vi "Version_2.0_Single_Column_Code.vi"() -> ()   [LabVIEW 2020] (continued)
                            n3570 = local read "VISA Refnum in\nfor Pump"() -> (w3951:refnum<visa-resource-name>)
                            n3571 = local read "Buffer-C2 Volume \nto be Pumped"() -> (w3947:dbl)
                            n3572 = local read "Volume of Syringe"() -> (w3950:dbl)
                            n3573 = call "RPickUp(SubVI).vi"("Volume to be picked up"=w3947, "Volume of Syringe"=w3950, "Resolution of PickUP"=w3948, "PickUp Flow Rate (ul/min)"=w3949, "VISA Refnum in"=w3951) -> ()  [unwired: 6 in, 1 out]
                            n3574 = local write "SEC On"(TRUE ("SEC On")) -> ()
                          }
                          frame #22 {
                            n3575 = local read "Stopper that ends \nthe main loops"() -> (w3952:bool)
                            n3576 = local read "VISA Refnum in\nfor Pump"() -> (w3953:refnum<visa-resource-name>)
                            n3577 = case shown="True" w3952 {
                              frame False {
                              }
                              frame True {
                                n3578 = local read "VISA Refnum in\nfor Pump"() -> (w3954:refnum<visa-resource-name>)
                                n3579 = call "HardStopCurrentProcess (SubVI).vi"("VISA Refnum in"=w3954) -> ()  [unwired: 11 in]
                              }
                            }
                            n3580 = call "ProcessCompletionWaiter (SubVI).vi"("VISA Refnum in"=w3953) -> ()  [unwired: 11 in]
                          }
                          frame #23 {
                            # "Reads the initial Plunger Position for computing the volume dispensed"
                            n3581 = local read "VISA Refnum in\nfor Pump"() -> (w3956:refnum<visa-resource-name>)
                            n3582 = call "AbsolutePlungerPosition (SubVI).vi"("VISA Refnum in"=w3956) -> ("Plunger Position"=w3955:i32)  [unwired: 10 in]
                            n3583 = local write "Initial Plunger Position"(w3955) -> ()
                          }
                          frame #24 {
                            # "Switch to Port-10"
                            # "Port-10 of the pump is conncted to column-2 of chip"
                            n3584 = local read "VISA Refnum in\nfor Pump"() -> (w3958:refnum<visa-resource-name>)
                            n3585 = call "PortChanger (SubVI).vi"("Port Number"="10", "VISA Refnum in"=w3958) -> ()  [unwired: 10 in]
                          }
                          frame #25 {
                            n3586 = local read "Stopper that ends \nthe main loops"() -> (w3959:bool)
                            n3587 = local read "VISA Refnum in\nfor Pump"() -> (w3960:refnum<visa-resource-name>)
                            n3588 = case shown="True" w3959 {
                              frame False {
                              }
                              frame True {
                                n3589 = local read "VISA Refnum in\nfor Pump"() -> (w3961:refnum<visa-resource-name>)
                                n3590 = call "HardStopCurrentProcess (SubVI).vi"("VISA Refnum in"=w3961) -> ()  [unwired: 11 in]
                              }
                            }
                            n3591 = call "ProcessCompletionWaiter (SubVI).vi"("VISA Refnum in"=w3960) -> ()  [unwired: 11 in]
                          }
                          frame #26 {
                            # "Keeps the AMF valve after column-1 open and valve after column-2 closed"
                            n3592 = local read "Buffer-C2 Dispense\nFlow Rate (ul/min)"() -> (w3974:dbl)
                            n3593 = local read "Buffer-C2 Pumping\nResolution"() -> (w3973:T2)
                            n3594 = local read "VISA Refnum in\nfor Pump"() -> (w3976:refnum<visa-resource-name>)
                            n3595 = local write "Pause Data Collection"(FALSE ("Pause Data Collection")) -> ()
                            n3596 = local read "Volume of Syringe"() -> (w3975:dbl)
                            n3597 = call "GoToAbsolutePosition(SubVI).vi"("Absolute Volume Position in Syringe (in ul)"=0.0 ("Volume to be Dispensed"), "Volume of Syringe"=w3975, "Resolution of Pumping"=w3973, "Flow Rate (ul/min)"=w3974, "VISA Refnum in"=w3976) -> ()  [unwired: 6 in, 1 out]
                            n3598 = local read "VISA Refnum in\nfor Valve"() -> (w3970:refnum<visa-resource-name>)
                            n3599 = local read "External Valve \nOPEN"() -> (w3969:string)
                            n3600 = local write "Valve V1 Open"(FALSE ("Valve V1 Open")) -> ()
                            n3601 = local write "Valve V2 Open"(TRUE ("Valve V2 Open")) -> ()
                            n3602 = local write "Valve V3 Open"(TRUE ("Valve V3 Open")) -> ()
                            n3603 = local write "Valve V4 Open"(FALSE ("Valve V4 Open")) -> ()
                            n3604 = call "PortChanger_Valve (SubVI).vi"("Port Number"=w3969, "VISA Refnum in"=w3970) -> ()  [unwired: 10 in]
                            n3605 = local write "Valve V5 Open"(FALSE ("Valve V5 Open")) -> ()
                            n3606 = local write "Valve V6 Open"(FALSE ("Valve V6 Open")) -> ()
                            n3607 = local write "Valve V7 Open"(FALSE ("Valve V7 Open")) -> ()
                          }
                          frame #27 {
                            n3608 = local read "Initial Plunger Position"() -> (w3980:dbl)
                            n3609 = local read "Buffer-C2 Pumping\nResolution"() -> (w3979:T2)
                            n3610 = local read "VISA Refnum in\nfor Pump"() -> (w3981:refnum<visa-resource-name>)
                            n3611 = local read "Volume of Syringe"() -> (w3978:dbl)
                            n3612 = while {
                              tunnel: w3980 -> [w3987]
                              tunnel: w3981 -> [w3986]
                              tunnel: w3979 -> [w3985]
                              tunnel: w3978 -> [w3984]
                              stop <- w3982 stop-if-true
                              n3613 = Wait (ms)(milliseconds to wait=u32 100) -> ()  [unwired: 1 out]
                              n3614 = stacked-sequence {
                                tunnel: w3987 -> [w3993 _]
                                tunnel: w3986 -> [w3992 w4019]
                                tunnel: w3985 -> [w3991 _]
                                tunnel: w3984 -> [w3990 _]
                                tunnel: [_ w4015] -> w3982
                                frame #0 {
                                n3615 = call "AbsolutePlungerPosition (SubVI).vi"("VISA Refnum in"=w3992) -> ("Plunger Position"=w3989:i32)  [unwired: 10 in]
                                n3616 = case shown="\"Standard Pumping\", Default" w3991 {
                                tunnel: w3993 -> [w3998 w4007]
                                tunnel: w3989 -> [w3999 w4006]
                                tunnel: [w3997 w4004] -> w3988
                                tunnel: w3990 -> [w3996 w4005]
                                frame "Standard Pumping", Default {
                                n3617 = Subtract(x=w3998, y=w3999) -> (x-y=w3995:dbl)
                                n3618 = Absolute Value(x=w3995) -> (abs(x)=w3994:dbl)
                                n3619 = Multiply(x=w3994, y=w3996) -> (x*y=w4001:dbl)
                                n3620 = Divide(x=w4001, y=3000.0) -> (x/y=w3997:dbl)
                                }
                                frame "High Resolution Pumping" {
                                n3621 = Subtract(x=w4007, y=w4006) -> (x-y=w4003:dbl)
                                n3622 = Absolute Value(x=w4003) -> (abs(x)=w4002:dbl)
                                n3623 = Multiply(x=w4002, y=w4005) -> (x*y=w4009:dbl)
                                n3624 = Divide(x=w4009, y=24000.0) -> (x/y=w4004:dbl)
                                }
                                }
                                n3625 = local write "Volume being Injected \nin this process"(w3988) -> ()
                                }
                                frame #1 {
                                n3626 = local read "Stopper that ends \nthe main loops"() -> (w4016:bool)
                                n3627 = local read "Divert Buffer-C \ninto Column-2"() -> (w4017:bool)
                                n3628 = local read "Volume being Injected \nin this process"() -> (w4014:dbl)
                                n3629 = call "LSPOneStatus (SubVI).vi"("VISA Refnum in"=w4019) -> ("read buffer"=w4021:string)  [unwired: 10 in]
                                n3630 = call <vilib>:"Trim Whitespace.vi"("string"=w4021) -> ("trimmed string"=w4020:string)  [unwired: 1 in]
                                n3631 = Equal?(x=w4020, y="/0`\u0003") -> (x = y?=w4018:bool)
                                n3632 = Or(x=w4017, y=w4016) -> (x .or. y?=w4012:bool)
                                n3633 = Greater Or Equal?(x=w4014, y=2.0) -> (x >= y?=w4011:bool)
                                n3634 = Or(x=w4012, y=w4011) -> (x .or. y?=w4010:bool)
                                n3635 = Or(x=w4018, y=w4010) -> (x .or. y?=w4015:bool)
                                }
                              }
                            }
                            n3636 = local read "Stopper that ends \nthe main loops"() -> (w3977:bool)
                            n3637 = case shown="True" w3977 {
                              frame False {
                              }
                              frame True {
                                n3638 = local read "VISA Refnum in\nfor Pump"() -> (w4023:refnum<visa-resource-name>)
                                n3639 = call "HardStopCurrentProcess (SubVI).vi"("VISA Refnum in"=w4023) -> ()  [unwired: 11 in]
                              }
                            }
                          }
                          frame #28 {
                            # "Keeps the on-chip valves V4, V5 and V7 open"
                            # "Keeps the AMF valve after column-1 closed and valve after column-2 open"
                            n3640 = local write "Divert Buffer-C \ninto Column-2"(FALSE ("Divert Buffer-C \ninto Column-2")) -> ()
                            n3641 = local read "VISA Refnum in\nfor Pump"() -> (w4028:refnum<visa-resource-name>)
                            n3642 = local read "External Valve \nCLOSED"() -> (w4027:string)
                            n3643 = local write "Valve V3 Open"(FALSE ("Valve V3 Open")) -> ()
                            n3644 = local write "Valve V2 Open"(FALSE ("Valve V2 Open")) -> ()
                            n3645 = local write "Valve V1 Open"(FALSE ("Valve V1 Open")) -> ()
                            n3646 = local write "Valve V4 Open"(TRUE ("Valve V4 Open")) -> ()
                            n3647 = call "PortChanger_Valve (SubVI).vi"("Port Number"=w4027, "VISA Refnum in"=w4028) -> ()  [unwired: 10 in]
                            n3648 = local write "Valve V5 Open"(TRUE ("Valve V5 Open")) -> ()
                            n3649 = local write "Valve V6 Open"(FALSE ("Valve V6 Open")) -> ()
                            n3650 = local write "Valve V7 Open"(TRUE ("Valve V7 Open")) -> ()
                          }
                          frame #29 {
                            n3651 = local read "Initial Plunger Position"() -> (w4037:dbl)
                            n3652 = local read "Buffer-C2 Pumping\nResolution"() -> (w4036:T2)
                            n3653 = local read "VISA Refnum in\nfor Pump"() -> (w4038:refnum<visa-resource-name>)
                            n3654 = local read "Volume of Syringe"() -> (w4035:dbl)
                            n3655 = while {
                              tunnel: w4037 -> [w4044]
                              tunnel: w4038 -> [w4043]
                              tunnel: w4036 -> [w4042]
                              tunnel: w4035 -> [w4041]
                              stop <- w4039 stop-if-true
                              n3656 = Wait (ms)(milliseconds to wait=u32 100) -> ()  [unwired: 1 out]
                              n3657 = stacked-sequence {
                                tunnel: w4044 -> [w4050 _]
                                tunnel: w4043 -> [w4049 w4072]
                                tunnel: w4042 -> [w4048 _]
                                tunnel: w4041 -> [w4047 _]
                                tunnel: [_ w4070] -> w4039
                                frame #0 {
                                n3658 = call "AbsolutePlungerPosition (SubVI).vi"("VISA Refnum in"=w4049) -> ("Plunger Position"=w4046:i32)  [unwired: 10 in]
                                n3659 = case shown="\"Standard Pumping\", Default" w4048 {
                                tunnel: w4050 -> [w4055 w4064]
                                tunnel: w4046 -> [w4056 w4063]
                                tunnel: [w4054 w4061] -> w4045
                                tunnel: w4047 -> [w4053 w4062]
                                frame "Standard Pumping", Default {
                                n3660 = Subtract(x=w4055, y=w4056) -> (x-y=w4052:dbl)
                                n3661 = Absolute Value(x=w4052) -> (abs(x)=w4051:dbl)
                                n3662 = Multiply(x=w4051, y=w4053) -> (x*y=w4058:dbl)
                                n3663 = Divide(x=w4058, y=3000.0) -> (x/y=w4054:dbl)
                                }
                                frame "High Resolution Pumping" {
                                n3664 = Subtract(x=w4064, y=w4063) -> (x-y=w4060:dbl)
                                n3665 = Absolute Value(x=w4060) -> (abs(x)=w4059:dbl)
                                n3666 = Multiply(x=w4059, y=w4062) -> (x*y=w4066:dbl)
                                n3667 = Divide(x=w4066, y=24000.0) -> (x/y=w4061:dbl)
                                }
                                }
                                n3668 = local write "Volume being Injected \nin this process"(w4045) -> ()
                                }
                                frame #1 {
                                n3669 = call "LSPOneStatus (SubVI).vi"("VISA Refnum in"=w4072) -> ("read buffer"=w4074:string)  [unwired: 10 in]
                                n3670 = call <vilib>:"Trim Whitespace.vi"("string"=w4074) -> ("trimmed string"=w4073:string)  [unwired: 1 in]
                                n3671 = Equal?(x=w4073, y="/0`\u0003") -> (x = y?=w4071:bool)
                                n3672 = local read "Stopper that ends \nthe main loops"() -> (w4068:bool)
                                n3673 = local read "Divert Sample \nonto Grid"() -> (w4069:bool)
                                n3674 = Or(x=w4069, y=w4068) -> (x .or. y?=w4067:bool)
                                n3675 = Or(x=w4071, y=w4067) -> (x .or. y?=w4070:bool)
                                }
                              }
                            }
                            n3676 = local read "Stopper that ends \nthe main loops"() -> (w4034:bool)
                            n3677 = case shown="True" w4034 {
                              frame False {
                              }
                              frame True {
                                n3678 = local read "VISA Refnum in\nfor Pump"() -> (w4076:refnum<visa-resource-name>)
                                n3679 = call "HardStopCurrentProcess (SubVI).vi"("VISA Refnum in"=w4076) -> ()  [unwired: 11 in]
                              }
                            }
                          }
                          frame #30 {
                            n3680 = local read "Volume being Injected \nin this process"() -> (w4079:dbl)
                            n3681 = local read "VISA Refnum in\nfor Pump"() -> (w4081:refnum<visa-resource-name>)
                            n3682 = call "AbsolutePlungerPosition (SubVI).vi"("VISA Refnum in"=w4081) -> ("Plunger Position"=w4080:i32)  [unwired: 10 in]
                            n3683 = local write "Pause Data Collection"(TRUE) -> ()
                            n3684 = local write "True Volume being \ninjected in this\nprocess"(w4079) -> ()
                            n3685 = local write "Position\nNow"(w4080) -> ()
                            n3686 = Wait (ms)(milliseconds to wait=u32 500) -> ()  [unwired: 1 out]
                          }
                          frame #31 {
                            # "Sample Deposition onto EM-Grid"
                            n3687 = local read "Divert Sample \nonto Grid"() -> (w4082:bool)
                            n3688 = case shown="True" w4082 {
                              frame False {
                              }
                              frame True {
                                n3689 = stacked-sequence {
                                frame #0 {
                                # "Discard the initial volume of fluid that is present in the channel prior to detection"
                                n3690 = local read "Buffer-C2 Pumping\nResolution"() -> (w4093:T2)
                                n3691 = local read "Initial Plunger Position"() -> (w4092:dbl)
                                n3692 = local read "VISA Refnum in\nfor Pump"() -> (w4094:refnum<visa-resource-name>)
                                n3693 = local read "Position\nNow"() -> (w4090:dbl)
                                n3694 = local read "Volume of Syringe"() -> (w4091:dbl)
                                n3695 = local write "Pause Data Collection"(FALSE) -> ()
                                n3696 = while {
                                tunnel: w4094 -> [w4104]
                                tunnel: w4093 -> [w4103]
                                tunnel: w4092 -> [w4099]
                                tunnel: w4091 -> [w4102]
                                tunnel: w4090 -> [w4098]
                                stop <- w4100 stop-if-true
                                n3697 = stacked-sequence {
                                tunnel: w4104 -> [w4110 w4132 w4162]
                                tunnel: w4103 -> [w4109 w4131 _]
                                tunnel: w4099 -> [w4107 _ _]
                                tunnel: w4102 -> [w4106 w4129 _]
                                tunnel: [_ _ w4155] -> w4100
                                tunnel: w4098 -> [_ w4127 _]
                                frame #0 {
                                # "From here on 'True Volume being injected \nin this process' represents the true total \nvolume in this process"
                                n3698 = call "AbsolutePlungerPosition (SubVI).vi"("VISA Refnum in"=w4110) -> ("Plunger Position"=w4108:i32)  [unwired: 10 in]
                                n3699 = case shown="..\"Standard Pumping\"" w4109 {
                                tunnel: w4108 -> [w4118 w4126]
                                tunnel: w4107 -> [w4117 w4125]
                                tunnel: w4106 -> [w4114 w4122]
                                tunnel: [w4111 w4119] -> w4105
                                frame .."Standard Pumping" {
                                n3700 = Subtract(x=w4118, y=w4117) -> (x-y=w4116:dbl)
                                n3701 = Absolute Value(x=w4116) -> (abs(x)=w4115:dbl)
                                n3702 = Multiply(x=w4115, y=w4114) -> (x*y=w4113:dbl)
                                n3703 = Divide(x=w4113, y=3000.0) -> (x/y=w4111:dbl)
                                }
                                frame "High Resolution Pumping".. {
                                n3704 = Subtract(x=w4126, y=w4125) -> (x-y=w4124:dbl)
                                n3705 = Absolute Value(x=w4124) -> (abs(x)=w4123:dbl)
                                n3706 = Multiply(x=w4123, y=w4122) -> (x*y=w4121:dbl)
                                n3707 = Divide(x=w4121, y=24000.0) -> (x/y=w4119:dbl)
                                }
                                }
                                n3708 = local write "True Volume being \ninjected in this\nprocess"(w4105) -> ()
                                }
                                frame #1 {
                                # "From here on 'Volume being injected \nin this process' represents the volume \nin this sub process"
                                n3709 = call "AbsolutePlungerPosition (SubVI).vi"("VISA Refnum in"=w4132) -> ("Plunger Position"=w4130:i32)  [unwired: 10 in]
                                n3710 = case shown="..\"Standard Pumping\"" w4131 {
                                tunnel: w4130 -> [w4140 w4148]
                                tunnel: w4127 -> [w4139 w4147]
                                tunnel: w4129 -> [w4136 w4144]
                                tunnel: [w4133 w4141] -> w4128
                                frame .."Standard Pumping" {
                                n3711 = Subtract(x=w4140, y=w4139) -> (x-y=w4138:dbl)
                                n3712 = Absolute Value(x=w4138) -> (abs(x)=w4137:dbl)
                                n3713 = Multiply(x=w4137, y=w4136) -> (x*y=w4135:dbl)
                                n3714 = Divide(x=w4135, y=3000.0) -> (x/y=w4133:dbl)
                                }
                                frame "High Resolution Pumping".. {
                                n3715 = Subtract(x=w4148, y=w4147) -> (x-y=w4146:dbl)
                                n3716 = Absolute Value(x=w4146) -> (abs(x)=w4145:dbl)
                                n3717 = Multiply(x=w4145, y=w4144) -> (x*y=w4143:dbl)
                                n3718 = Divide(x=w4143, y=24000.0) -> (x/y=w4141:dbl)
                                }
                                }
                                n3719 = local write "Volume being Injected \nin this process"(w4128) -> ()
                                }
                                frame #2 {
                                n3720 = local read "Discard Volume"() -> (w4149:dbl)
                                n3721 = local read "Discard fluid \nprior to 1st \ndeposition"() -> (w4154:bool)
                                n3722 = local read "Volume being Injected \nin this process"() -> (w4153:dbl)
                                n3723 = Greater Or Equal?(x=w4153, y=w4149) -> (x >= y?=w4151:bool)
                                n3724 = call "AbsolutePlungerPositionStatus (SubVI).vi"("VISA Refnum in"=w4162) -> ("read buffer"=w4161:string)  [unwired: 10 in]
                                n3725 = local read "Stop for End of \nExperiment \nand Data Writing"() -> (w4158:bool)
                                n3726 = call <vilib>:"Trim Whitespace.vi"("string"=w4161) -> ("trimmed string"=w4160:string)  [unwired: 1 in]
                                n3727 = Not(x=w4154) -> (.not. x?=w4152:bool)
                                n3728 = Equal?(x=w4160, y="/0`\u0003") -> (x = y?=w4157:bool)
                                n3729 = Or(x=w4152, y=w4151) -> (x .or. y?=w4150:bool)
                                n3730 = Or(x=w4150, y=w4158) -> (x .or. y?=w4156:bool)
                                n3731 = Or(x=w4157, y=w4156) -> (x .or. y?=w4155:bool)
                                }
                                }
                                n3732 = Wait (ms)(milliseconds to wait=u32 100) -> ()  [unwired: 1 out]
                                }
                                n3733 = local write "Valve V4 Open"(TRUE ("Valve V4 Open")) -> ()
                                n3734 = local write "Valve V3 Open"(FALSE ("Valve V3 Open")) -> ()
                                n3735 = local write "Valve V2 Open"(FALSE ("Valve V2 Open")) -> ()
                                n3736 = local write "Valve V1 Open"(FALSE ("Valve V1 Open")) -> ()
                                n3737 = local write "Valve V5 Open"(TRUE ("Valve V5 Open")) -> ()
                                n3738 = local write "Valve V6 Open"(TRUE ("Valve V6 Open")) -> ()
                                n3739 = local write "Valve V7 Open"(FALSE ("Valve V7 Open")) -> ()
                                n3740 = local write "Volume being Injected \nin this process"(0.0) -> ()
                                }
                                frame #1 {
                                # "Keeps the on-chip valve V1, V2 and V3 closed,\nHalts also deposition onto the grid\nand waits for the 1st redeposit command. Once the command is issued\nit starts pumpoing and moves onto the next frame"
                                n3741 = stacked-sequence {
                                frame #0 {
                                n3742 = local write "Valve V5 Open"(FALSE ("Valve V5 Open")) -> ()
                                n3743 = local write "Valve V1 Open"(FALSE ("Valve V1 Open")) -> ()
                                n3744 = local read "VISA Refnum in\nfor Pump"() -> (w4172:refnum<visa-resource-name>)
                                n3745 = local write "Valve V2 Open"(FALSE ("Valve V2 Open")) -> ()
                                n3746 = local write "Valve V6 Open"(FALSE ("Valve V6 Open")) -> ()
                                n3747 = local write "Re-deposit Sample\nonto Grid"(FALSE ("Redeposit Sample\nonto Grid")) -> ()
                                n3748 = local write "Pause Data Collection"(TRUE ("Pause Data Collection")) -> ()
                                n3749 = call "HardStopCurrentProcess (SubVI).vi"("VISA Refnum in"=w4172) -> ()  [unwired: 11 in]
                                n3750 = local write "Valve V7 Open"(FALSE ("Valve V7 Open")) -> ()
                                n3751 = local write "Valve V3 Open"(FALSE ("Valve V3 Open")) -> ()
                                n3752 = local write "Valve V4 Open"(FALSE ("Valve V4 Open")) -> ()
                                }
                                frame #1 {
                                n3753 = while {
                                stop <- w4175 stop-if-true
                                n3754 = local read "Stop for End of \nExperiment \nand Data Writing"() -> (w4176:bool)
                                n3755 = local read "Re-deposit Sample\nonto Grid"() -> (w4177:bool)
                                n3756 = Or(x=w4177, y=w4176) -> (x .or. y?=w4175:bool)
                                }
                                n3757 = local write "Discard fluid \nprior to 1st \ndeposition"(FALSE ("Discard fluid \nprior to 1st \ndeposition")) -> ()
                                n3758 = One Button Dialog(message="Do you want to deposit sample on another grid? If yes, turn on 'Re-deposit Sample onto Grid'. Else turn on STOP ") -> ()  [unwired: 1 in, 1 out]
                                }
                                frame #2 {
                                n3759 = local write "Valve V6 Open"(TRUE ("Valve V3 Open")) -> ()
                                n3760 = local write "Valve V4 Open"(TRUE ("Valve V1 Open")) -> ()
                                n3761 = local write "Valve V5 Open"(TRUE ("Valve V2 Open")) -> ()
                                n3762 = local write "Valve V7 Open"(FALSE ("Valve V7 Open")) -> ()
                                }
                                frame #3 {
                                n3763 = local read "Re-deposit Sample\nonto Grid"() -> (w4182:bool)
                                n3764 = case shown="True" w4182 {
                                frame False {
                                n3765 = local write "Suction On/Off"(FALSE ("Suction On/Off")) -> ()
                                }
                                frame True {
                                n3766 = stacked-sequence {
                                frame #0 {
                                n3767 = local read "VISA Refnum in\nfor Pump"() -> (w4185:refnum<visa-resource-name>)
                                n3768 = call "AbsolutePlungerPosition (SubVI).vi"("VISA Refnum in"=w4185) -> ("Plunger Position"=w4184:i32)  [unwired: 10 in]
                                n3769 = local write "Position\nNow"(w4184) -> ()
                                }
                                frame #1 {
                                n3770 = local read "Buffer-C2 Pumping\nResolution"() -> (w4187:T2)
                                n3771 = case shown="\"Standard Pumping\", Default" w4187 {
                                tunnel: [w4188 w4199] -> w4186
                                frame "Standard Pumping", Default {
                                n3772 = local read "Buffer-C2 Volume \nto be Pumped"() -> (w4191:dbl)
                                n3773 = local read "Volume of Syringe"() -> (w4194:dbl)
                                n3774 = local read "Initial Plunger Position"() -> (w4198:dbl)
                                n3775 = local read "Position\nNow"() -> (w4197:dbl)
                                n3776 = Subtract(x=w4198, y=w4197) -> (x-y=w4196:dbl)
                                n3777 = Absolute Value(x=w4196) -> (abs(x)=w4195:dbl)
                                n3778 = Multiply(x=w4195, y=w4194) -> (x*y=w4193:dbl)
                                n3779 = Divide(x=w4193, y=3000.0) -> (x/y=w4190:dbl)
                                n3780 = Subtract(x=w4190, y=w4191) -> (x-y=w4189:dbl)
                                n3781 = Absolute Value(x=w4189) -> (abs(x)=w4188:dbl)
                                }
                                frame "High Resolution Pumping" {
                                n3782 = local read "Buffer-C2 Volume \nto be Pumped"() -> (w4202:dbl)
                                n3783 = local read "Volume of Syringe"() -> (w4205:dbl)
                                n3784 = local read "Initial Plunger Position"() -> (w4209:dbl)
                                n3785 = local read "Position\nNow"() -> (w4208:dbl)
                                n3786 = Subtract(x=w4209, y=w4208) -> (x-y=w4207:dbl)
                                n3787 = Absolute Value(x=w4207) -> (abs(x)=w4206:dbl)
                                n3788 = Multiply(x=w4206, y=w4205) -> (x*y=w4204:dbl)
                                n3789 = Divide(x=w4204, y=24000.0) -> (x/y=w4201:dbl)
                                n3790 = Subtract(x=w4201, y=w4202) -> (x-y=w4200:dbl)
                                n3791 = Absolute Value(x=w4200) -> (abs(x)=w4199:dbl)
                                }
                                }
                                n3792 = local write "Buffer-C Volume\nleft to be Pumped"(w4186) -> ()
                                }
                                frame #2 {
                                n3793 = local read "Buffer-C2 Dispense\nFlow Rate (ul/min)"() -> (w4213:dbl)
                                n3794 = local read "Buffer-C2 Pumping\nResolution"() -> (w4212:T2)
                                n3795 = local read "VISA Refnum in\nfor Pump"() -> (w4215:refnum<visa-resource-name>)
                                n3796 = local read "Volume of Syringe"() -> (w4214:dbl)
                                n3797 = call "GoToAbsolutePosition(SubVI).vi"("Absolute Volume Position in Syringe (in ul)"=0.0, "Volume of Syringe"=w4214, "Resolution of Pumping"=w4212, "Flow Rate (ul/min)"=w4213, "VISA Refnum in"=w4215) -> ()  [unwired: 6 in, 1 out]
                                n3798 = local write "Suction On/Off"(FALSE ("Suction On/Off")) -> ()
                                }
                                }
                                }
                                }
                                }
                                frame #4 {
                                n3799 = local read "Stop for End of \nExperiment \nand Data Writing"() -> (w4216:bool)
                                n3800 = case shown="True" w4216 {
                                frame False {
                                }
                                frame True {
                                n3801 = local read "VISA Refnum in\nfor Pump"() -> (w4217:refnum<visa-resource-name>)
                                n3802 = call "HardStopCurrentProcess (SubVI).vi"("VISA Refnum in"=w4217) -> ()  [unwired: 11 in]
                                }
                                }
                                }
                                }
                                }
                                frame #2 {
                                # "Keeps the on-chip valve V1, V2 Open and V3 closed"
                                n3803 = while {
                                stop <- w4221 stop-if-true
                                n3804 = local read "Suction On/Off"() -> (w4222:bool)
                                n3805 = case shown="True" w4222 {
                                frame False {
                                n3806 = local read "Buffer-C2 Pumping\nResolution"() -> (w4228:T2)
                                n3807 = local read "Initial Plunger Position"() -> (w4227:dbl)
                                n3808 = local read "VISA Refnum in\nfor Pump"() -> (w4229:refnum<visa-resource-name>)
                                n3809 = local read "Position\nNow"() -> (w4225:dbl)
                                n3810 = local read "Volume of Syringe"() -> (w4226:dbl)
                                n3811 = local write "Volume being Injected \nin this process"(0.0) -> ()
                                n3812 = local write "Pause Data Collection"(FALSE) -> ()
                                n3813 = while {
                                tunnel: w4229 -> [w4236]
                                tunnel: w4228 -> [w4235]
                                tunnel: w4227 -> [w4231]
                                tunnel: w4226 -> [w4234]
                                tunnel: w4225 -> [w4230]
                                stop <- w4232 stop-if-true
                                n3814 = stacked-sequence {
                                tunnel: w4236 -> [w4242 w4264 w4289]
                                tunnel: w4235 -> [w4241 w4263 _]
                                tunnel: w4231 -> [w4239 _ _]
                                tunnel: w4234 -> [w4238 w4261 _]
                                tunnel: [_ _ w4281] -> w4232
                                tunnel: w4230 -> [_ w4259 _]
                                frame #0 {
                                # "From here on 'True Volume being injected \nin this process' represents the true total \nvolume in this process"
                                n3815 = call "AbsolutePlungerPosition (SubVI).vi"("VISA Refnum in"=w4242) -> ("Plunger Position"=w4240:i32)  [unwired: 10 in]
                                n3816 = case shown="..\"Standard Pumping\"" w4241 {
                                tunnel: w4240 -> [w4250 w4258]
                                tunnel: w4239 -> [w4249 w4257]
                                tunnel: w4238 -> [w4246 w4254]
                                tunnel: [w4243 w4251] -> w4237
                                frame .."Standard Pumping" {
                                n3817 = Subtract(x=w4250, y=w4249) -> (x-y=w4248:dbl)
                                n3818 = Absolute Value(x=w4248) -> (abs(x)=w4247:dbl)
                                n3819 = Multiply(x=w4247, y=w4246) -> (x*y=w4245:dbl)
                                n3820 = Divide(x=w4245, y=3000.0) -> (x/y=w4243:dbl)
                                }
                                frame "High Resolution Pumping".. {
                                n3821 = Subtract(x=w4258, y=w4257) -> (x-y=w4256:dbl)
                                n3822 = Absolute Value(x=w4256) -> (abs(x)=w4255:dbl)
                                n3823 = Multiply(x=w4255, y=w4254) -> (x*y=w4253:dbl)
                                n3824 = Divide(x=w4253, y=24000.0) -> (x/y=w4251:dbl)
                                }
                                }
                                n3825 = local write "True Volume being \ninjected in this\nprocess"(w4237) -> ()
                                }
                                frame #1 {
                                # "From here on 'Volume being injected \nin this process' represents the volume \nin this sub process"
                                n3826 = call "AbsolutePlungerPosition (SubVI).vi"("VISA Refnum in"=w4264) -> ("Plunger Position"=w4262:i32)  [unwired: 10 in]
                                n3827 = case shown="..\"Standard Pumping\"" w4263 {
                                tunnel: w4262 -> [w4272 w4280]
                                tunnel: w4259 -> [w4271 w4279]
                                tunnel: w4261 -> [w4268 w4276]
                                tunnel: [w4265 w4273] -> w4260
                                frame .."Standard Pumping" {
                                n3828 = Subtract(x=w4272, y=w4271) -> (x-y=w4270:dbl)
                                n3829 = Absolute Value(x=w4270) -> (abs(x)=w4269:dbl)
                                n3830 = Multiply(x=w4269, y=w4268) -> (x*y=w4267:dbl)
                                n3831 = Divide(x=w4267, y=3000.0) -> (x/y=w4265:dbl)
                                }
                                frame "High Resolution Pumping".. {
                                n3832 = Subtract(x=w4280, y=w4279) -> (x-y=w4278:dbl)
                                n3833 = Absolute Value(x=w4278) -> (abs(x)=w4277:dbl)
                                n3834 = Multiply(x=w4277, y=w4276) -> (x*y=w4275:dbl)
                                n3835 = Divide(x=w4275, y=24000.0) -> (x/y=w4273:dbl)
                                }
                                }
                                n3836 = local write "Volume being Injected \nin this process"(w4260) -> ()
                                }
                                frame #2 {
                                n3837 = local read "Stop for End of \nExperiment \nand Data Writing"() -> (w4284:bool)
                                n3838 = local read "Suction On/Off"() -> (w4285:bool)
                                n3839 = call "AbsolutePlungerPositionStatus (SubVI).vi"("VISA Refnum in"=w4289) -> ("read buffer"=w4288:string)  [unwired: 10 in]
                                n3840 = call <vilib>:"Trim Whitespace.vi"("string"=w4288) -> ("trimmed string"=w4287:string)  [unwired: 1 in]
                                n3841 = Equal?(x=w4287, y="/0`\u0003") -> (x = y?=w4283:bool)
                                n3842 = Or(x=w4285, y=w4284) -> (x .or. y?=w4282:bool)
                                n3843 = Or(x=w4283, y=w4282) -> (x .or. y?=w4281:bool)
                                }
                                }
                                n3844 = Wait (ms)(milliseconds to wait=u32 100) -> ()  [unwired: 1 out]
                                }
                                }
                                frame True {
                                n3845 = stacked-sequence {
                                frame #0 {
                                n3846 = local read "Suction Pressure\nfor EM-grid \nDeposition (mbar)"() -> (w4294:sgl)
                                n3847 = local write "Valve V4 Open"(FALSE ("Valve V4 Open")) -> ()
                                n3848 = local read "VISA Refnum in\nfor Pump"() -> (w4297:refnum<visa-resource-name>)
                                n3849 = local write "Valve V5 Open"(FALSE ("Valve V1 Open")) -> ()
                                n3850 = local write "Suction pressure \nfor grid deposition"(w4294) -> ()
                                n3851 = local write "Re-deposit Sample\nonto Grid"(FALSE ("Redeposit Sample\nonto Grid")) -> ()
                                n3852 = local write "Pause Data Collection"(TRUE ("Pause Data Collection")) -> ()
                                n3853 = call "HardStopCurrentProcess (SubVI).vi"("VISA Refnum in"=w4297) -> ()  [unwired: 11 in]
                                n3854 = local write "Valve V6 Open"(TRUE ("Valve V2 Open")) -> ()
                                n3855 = local write "Valve V7 Open"(TRUE ("Valve V3 Open")) -> ()
                                }
                                frame #1 {
                                n3856 = call <vilib>:"fgt init.vi"() -> ("error out"=w4298:errorcluster)  [unwired: 11 in]
                                n3857 = while {
                                tunnel: [w4302] -> w4299
                                tunnel: w4298 -> [w4301]
                                stop <- w4305 stop-if-true
                                # "'5' corresponds to 2nd positin in the line-up series"
                                n3858 = local read "Suction On/Off"() -> (w4300:bool)
                                n3859 = local read "Stop for End of \nExperiment \nand Data Writing"() -> (w4306:bool)
                                n3860 = case shown="True" w4300 {
                                tunnel: [0 w4311] -> w4303
                                frame False {
                                }
                                frame True {
                                n3861 = local read "Suction Pressure\nfor EM-grid \nDeposition (mbar)"() -> (w4311:sgl)
                                }
                                }
                                n3862 = call <vilib>:"fgt set pressure.vi"("error in (no error)"=w4301, "pressure"=w4303, "pressureIndex"=u32 1) -> ("error out"=w4302:errorcluster)  [unwired: 8 in]
                                n3863 = local read "Suction On/Off"() -> (w4308:bool)
                                n3864 = Not(x=w4308) -> (.not. x?=w4307:bool)
                                n3865 = Wait (ms)(milliseconds to wait=u32 100) -> ()  [unwired: 1 out]
                                n3866 = Or(x=w4307, y=w4306) -> (x .or. y?=w4305:bool)
                                }
                                n3867 = call <vilib>:"fgt close.vi"("error in (no error)"=w4299) -> ()  [unwired: 10 in, 1 out]
                                }
                                frame #2 {
                                n3868 = local write "Valve V7 Open"(FALSE ("Valve V3 Open")) -> ()
                                n3869 = local write "Valve V5 Open"(FALSE ("Valve V1 Open")) -> ()
                                n3870 = local write "Valve V6 Open"(FALSE ("Valve V2 Open")) -> ()
                                n3871 = local write "Valve V4 Open"(FALSE ("Valve V4 Open")) -> ()
                                }
                                frame #3 {
                                n3872 = while {
                                stop <- w4317 stop-if-true
                                n3873 = local read "Stop for End of \nExperiment \nand Data Writing"() -> (w4318:bool)
                                n3874 = local read "Re-deposit Sample\nonto Grid"() -> (w4319:bool)
                                n3875 = Or(x=w4319, y=w4318) -> (x .or. y?=w4317:bool)
                                }
                                n3876 = One Button Dialog(message="Do you want to deposit sample on another grid? If yes, turn on 'Re-deposit Sample onto Grid'. Else turn on STOP ") -> ()  [unwired: 1 in, 1 out]
                                }
                                frame #4 {
                                n3877 = local write "Valve V4 Open"(TRUE ("Valve V4 Open")) -> ()
                                n3878 = local write "Valve V7 Open"(FALSE ("Valve V3 Open")) -> ()
                                n3879 = local write "Valve V5 Open"(TRUE ("Valve V1 Open")) -> ()
                                n3880 = local write "Valve V6 Open"(TRUE ("Valve V2 Open")) -> ()
                                }
                                frame #5 {
                                n3881 = local read "Re-deposit Sample\nonto Grid"() -> (w4324:bool)
                                n3882 = case shown="False" w4324 {
                                frame False {
                                n3883 = local write "Suction On/Off"(FALSE ("Suction On/Off")) -> ()
                                }
                                frame True {
                                n3884 = stacked-sequence {
                                frame #0 {
                                n3885 = local read "VISA Refnum in\nfor Pump"() -> (w4327:refnum<visa-resource-name>)
                                n3886 = call "AbsolutePlungerPosition (SubVI).vi"("VISA Refnum in"=w4327) -> ("Plunger Position"=w4326:i32)  [unwired: 10 in]
                                n3887 = local write "Position\nNow"(w4326) -> ()
                                }
                                frame #1 {
                                n3888 = local read "Buffer-C2 Pumping\nResolution"() -> (w4329:T2)
                                n3889 = case shown="\"Standard Pumping\", Default" w4329 {
                                tunnel: [w4330 w4341] -> w4328
                                frame "Standard Pumping", Default {
                                n3890 = local read "Buffer-C2 Volume \nto be Pumped"() -> (w4333:dbl)
                                n3891 = local read "Volume of Syringe"() -> (w4336:dbl)
                                n3892 = local read "Initial Plunger Position"() -> (w4340:dbl)
                                n3893 = local read "Position\nNow"() -> (w4339:dbl)
                                n3894 = Subtract(x=w4340, y=w4339) -> (x-y=w4338:dbl)
                                n3895 = Absolute Value(x=w4338) -> (abs(x)=w4337:dbl)
                                n3896 = Multiply(x=w4337, y=w4336) -> (x*y=w4335:dbl)
                                n3897 = Divide(x=w4335, y=3000.0) -> (x/y=w4332:dbl)
                                n3898 = Subtract(x=w4332, y=w4333) -> (x-y=w4331:dbl)
                                n3899 = Absolute Value(x=w4331) -> (abs(x)=w4330:dbl)
                                }
                                frame "High Resolution Pumping" {
                                n3900 = local read "Buffer-C2 Volume \nto be Pumped"() -> (w4344:dbl)
                                n3901 = local read "Volume of Syringe"() -> (w4347:dbl)
                                n3902 = local read "Initial Plunger Position"() -> (w4351:dbl)
                                n3903 = local read "Position\nNow"() -> (w4350:dbl)
                                n3904 = Subtract(x=w4351, y=w4350) -> (x-y=w4349:dbl)
                                n3905 = Absolute Value(x=w4349) -> (abs(x)=w4348:dbl)
                                n3906 = Multiply(x=w4348, y=w4347) -> (x*y=w4346:dbl)
                                n3907 = Divide(x=w4346, y=24000.0) -> (x/y=w4343:dbl)
                                n3908 = Subtract(x=w4343, y=w4344) -> (x-y=w4342:dbl)
                                n3909 = Absolute Value(x=w4342) -> (abs(x)=w4341:dbl)
                                }
                                }
                                n3910 = local write "Buffer-C Volume\nleft to be Pumped"(w4328) -> ()
                                }
                                frame #2 {
                                n3911 = local read "Buffer-C2 Dispense\nFlow Rate (ul/min)"() -> (w4355:dbl)
                                n3912 = local read "Buffer-C2 Pumping\nResolution"() -> (w4354:T2)
                                n3913 = local read "VISA Refnum in\nfor Pump"() -> (w4357:refnum<visa-resource-name>)
                                n3914 = local read "Volume of Syringe"() -> (w4356:dbl)
                                n3915 = call "GoToAbsolutePosition(SubVI).vi"("Absolute Volume Position in Syringe (in ul)"=0.0, "Volume of Syringe"=w4356, "Resolution of Pumping"=w4354, "Flow Rate (ul/min)"=w4355, "VISA Refnum in"=w4357) -> ()  [unwired: 6 in, 1 out]
                                n3916 = local write "Suction On/Off"(FALSE ("Suction On/Off")) -> ()
                                }
                                }
                                }
                                }
                                }
                                frame #6 {
                                n3917 = local read "Stop for End of \nExperiment \nand Data Writing"() -> (w4358:bool)
                                n3918 = case shown="True" w4358 {
                                frame False {
                                }
                                frame True {
                                n3919 = local read "VISA Refnum in\nfor Pump"() -> (w4359:refnum<visa-resource-name>)
                                n3920 = call "HardStopCurrentProcess (SubVI).vi"("VISA Refnum in"=w4359) -> ()  [unwired: 11 in]
                                }
                                }
                                }
                                }
                                }
                                }
                                n3921 = local read "Stop for End of \nExperiment \nand Data Writing"() -> (w4220:bool)
                                n3922 = local read "Divert Sample \nonto Grid"() -> (w4219:bool)
                                n3923 = Not(x=w4219) -> (.not. x?=w4218:bool)
                                n3924 = Or(x=w4218, y=w4220) -> (x .or. y?=w4221:bool)
                                }
                                }
                                }
                                n3925 = local write "Discard fluid \nprior to 1st \ndeposition"(TRUE ("Discard fluid \nprior to 1st \ndeposition")) -> ()
                              }
                            }
                          }
                          frame #32 {
                            n3926 = local write "Valve V2 Open"(FALSE ("Valve V2 Open")) -> ()
                            n3927 = local write "Valve V4 Open"(FALSE ("Valve V4 Open")) -> ()
                            n3928 = local write "Valve V3 Open"(FALSE ("Valve V3 Open")) -> ()
                            n3929 = local write "Valve V1 Open"(FALSE ("Valve V1 Open")) -> ()
                            n3930 = local write "Valve V6 Open"(FALSE ("Valve V6 Open")) -> ()
                            n3931 = local write "Valve V5 Open"(FALSE ("Valve V5 Open")) -> ()
                            n3932 = local write "Valve V7 Open"(FALSE ("Valve V7 Open")) -> ()
                            n3933 = local read "VISA Refnum in\nfor Valve"() -> (w4364:refnum<visa-resource-name>)
                            n3934 = local read "External Valve \nOPEN"() -> (w4363:string)
                            n3935 = Wait (ms)(milliseconds to wait=u32 500) -> ()  [unwired: 1 out]
                            n3936 = call "PortChanger_Valve (SubVI).vi"("Port Number"=w4363, "VISA Refnum in"=w4364) -> ()  [unwired: 10 in]
                          }
                          frame #33 {
                            n3937 = local read "Stopper that ends \nthe main loops"() -> (w4371:bool)
                            n3938 = Wait (ms)(milliseconds to wait=u32 500) -> ()  [unwired: 1 out]
                            n3939 = case shown="True" w4371 {
                              frame False {
                              }
                              frame True {
                                n3940 = local read "VISA Refnum in\nfor Pump"() -> (w4375:refnum<visa-resource-name>)
                                n3941 = call "HardStopCurrentProcess (SubVI).vi"("VISA Refnum in"=w4375) -> ()  [unwired: 11 in]
                              }
                            }
                            n3942 = local write "Pause Data Collection"(TRUE ("Pause Data Collection")) -> ()
                            n3943 = local write "Start the Process"(FALSE ("Start the Process")) -> ()
                            n3944 = local write "Divert Sample \nonto Grid"(FALSE ("Divert Sample \nonto Grid")) -> ()
                          }
                          frame #34 {
                            n3945 = local write "Volume being Injected \nin this process"(0.0 ("Volume being Injected \nin this process")) -> ()
                            n3946 = local write "Elution of Column-2"(FALSE ("Elution of Column-2")) -> ()
                            n3947 = local write "SEC On"(FALSE ("SEC On")) -> ()
                          }
                        }
                      }
                    }
                  }
                }
              }
              frame True {
                n3948 = local write "Pause Data Collection"(FALSE ("Pause Data Collection")) -> ()
              }
            }
          }
          frame "Automated Protein Purification with Re-SEC Possibility, 8 SOD Valves and On/Off External Valve" {
            n3949 = local read "Stopper that ends \nthe main loops"() -> (w4380:bool)
            n3950 = case shown="False" w4380 {
              frame False {
                n3951 = local read "Start the Process"() -> (w4381:bool)
                n3952 = case shown="True" w4381 {
                  frame False {
                    n3953 = local read "Stopper that ends \nthe main loops"() -> (w4383:bool)
                    n3954 = local read "Start the Process"() -> (w4382:bool)
                    n3955 = Or(x=w4383, y=w4382) -> (x .or. y?=w4384:bool)
                    n3956 = case shown="False" w4384 {
                      frame False {
                        n3957 = while {
                          stop <- w4387 stop-if-true
                          n3958 = local read "Stop for End of \nExperiment \nand Data Writing"() -> (w4386:bool)
                          n3959 = local read "Stopper that ends \nthe main loops"() -> (w4389:bool)
                          n3960 = local read "Start the Process"() -> (w4388:bool)
                          n3961 = Wait (ms)(milliseconds to wait=u32 10) -> ()  [unwired: 1 out]
                          n3962 = Or(x=w4389, y=w4388) -> (x .or. y?=w4387:bool)
                          n3963 = local write "Stopper that ends \nthe main loops"(w4386) -> ()
                        }
                        n3964 = One Button Dialog(message="Please Select the Process and Press 'Start the Process' Button") -> ()  [unwired: 1 in, 1 out]
                      }
                      frame True {
                      }
                    }
                  }
                  frame True {
                    n3965 = stacked-sequence {
                      frame #0 {
                        # "Equilibrate Column-1 with Buffer-A obtained from port-4 and pumped via port-2 and Column-2 with Buffer-C obtained from port-4 and pumped onto chip via port-6 onto the chip ...with an initial and inbetween wash of tubings while changing the buffers"
                        n3966 = stacked-sequence {
                          frame #0 {
                            n3967 = local write "Equilibriating \nColumn-1"(TRUE ("Equilibriating \nColumn-1")) -> ()
                            n3968 = local write "External Valve \nOpen"(FALSE ("External Valve \nOpen")) -> ()
                            n3969 = local write "Valve V4 Open"(FALSE ("Valve V4 Open")) -> ()
                            n3970 = local write "Valve V1 Open"(FALSE ("Valve V1 Open")) -> ()
                            n3971 = local write "Valve V2 Open"(FALSE ("Valve V2 Open")) -> ()
                            n3972 = local write "Valve V3 Open"(FALSE ("Valve V3 Open")) -> ()
                            n3973 = local write "Valve V7 Open"(FALSE ("Valve V7 Open")) -> ()
                            n3974 = local write "Valve V8 Open"(FALSE ("Valve V8 Open")) -> ()
                            n3975 = local write "Valve V5 Open"(FALSE ("Valve V5 Open")) -> ()
                            n3976 = local write "Valve V6 Open"(FALSE ("Valve V6 Open")) -> ()
                            n3977 = call <vilib>:"fgt init.vi"() -> ("error out"=w4395:errorcluster)  [unwired: 11 in]
                            n3978 = while {
                              tunnel: w4395 -> [w4404]
                              tunnel: [w4403] -> w4394
                              stop <- w4407 stop-if-true
                              # "Keeping the valve closing pressure of push pull to zero"
                              n3979 = local read "Stop for End of \nExperiment \nand Data Writing"() -> (w4408:bool)
                              n3980 = local read "Equilibriating \nColumn-1"() -> (w4409:bool)
                              n3981 = call <vilib>:"fgt set pressure.vi"("error in (no error)"=w4404, "pressure"=sgl 0.0 ("order"), "pressureIndex"=1 ("module")) -> ("error out"=w4403:errorcluster)  [unwired: 8 in]
                              n3982 = Or(x=w4409, y=w4408) -> (x .or. y?=w4407:bool)
                              n3983 = Wait (ms)(milliseconds to wait=u32 10) -> ()  [unwired: 1 out]
                            }
                            n3984 = call <vilib>:"fgt close.vi"("error in (no error)"=w4394) -> ()  [unwired: 10 in, 1 out]
                          }
                          frame #1 {
                            # "Clean the elution tubing with Buffer-B1"
                            n3985 = local read "N-B1"() -> (w4411:i32)
                            n3986 = for {
                              N: w4411 -> [_]
                              n3987 = stacked-sequence {
                                frame #0 {
                                n3988 = local read "VISA Refnum in\nfor Pump"() -> (w4414:refnum<visa-resource-name>)
                                n3989 = local read "Port for \nB-Elution"() -> (w4413:string)
                                n3990 = call "PortChanger (SubVI).vi"("Port Number"=w4413, "VISA Refnum in"=w4414) -> ()  [unwired: 10 in]
                                }
                                frame #1 {
                                n3991 = local read "VISA Refnum in\nfor Pump"() -> (w4415:refnum<visa-resource-name>)
                                n3992 = call "ProcessCompletionWaiter (SubVI).vi"("VISA Refnum in"=w4415) -> ()  [unwired: 11 in]
                                }
                                frame #2 {
                                n3993 = local read "VISA Refnum in\nfor Pump"() -> (w4420:refnum<visa-resource-name>)
                                n3994 = local read "Apparent Volume\nof Syringe"() -> (w4416:dbl)
                                n3995 = local read "Volume of Syringe"() -> (w4417:dbl)
                                n3996 = call "RPickUp(SubVI).vi"("Volume to be picked up"=w4416, "Volume of Syringe"=w4417, "Resolution of PickUP"=T2."Standard Pumping", "PickUp Flow Rate (ul/min)"=150.0, "VISA Refnum in"=w4420) -> ()  [unwired: 6 in, 1 out]
                                }
                                frame #3 {
                                n3997 = local read "Stopper that ends \nthe main loops"() -> (w4421:bool)
                                n3998 = local read "VISA Refnum in\nfor Pump"() -> (w4422:refnum<visa-resource-name>)
                                n3999 = case shown="True" w4421 {
                                frame False {
                                }
                                frame True {
                                n4000 = local read "VISA Refnum in\nfor Pump"() -> (w4423:refnum<visa-resource-name>)
                                n4001 = call "HardStopCurrentProcess (SubVI).vi"("VISA Refnum in"=w4423) -> ()  [unwired: 11 in]
                                }
                                }
                                n4002 = call "ProcessCompletionWaiter (SubVI).vi"("VISA Refnum in"=w4422) -> ()  [unwired: 11 in]
                                }
                                frame #4 {
                                n4003 = local read "VISA Refnum in\nfor Pump"() -> (w4425:refnum<visa-resource-name>)
                                n4004 = call "PortChanger (SubVI).vi"("Port Number"="1", "VISA Refnum in"=w4425) -> ()  [unwired: 10 in]
                                }
                                frame #5 {
                                n4005 = local read "Stopper that ends \nthe main loops"() -> (w4426:bool)
                                n4006 = local read "VISA Refnum in\nfor Pump"() -> (w4427:refnum<visa-resource-name>)
                                n4007 = case shown="True" w4426 {
                                frame False {
                                }
                                frame True {
                                n4008 = local read "VISA Refnum in\nfor Pump"() -> (w4428:refnum<visa-resource-name>)
                                n4009 = call "HardStopCurrentProcess (SubVI).vi"("VISA Refnum in"=w4428) -> ()  [unwired: 11 in]
                                }
                                }
                                n4010 = call "ProcessCompletionWaiter (SubVI).vi"("VISA Refnum in"=w4427) -> ()  [unwired: 11 in]
                                }
                                frame #6 {
                                n4011 = local read "VISA Refnum in\nfor Pump"() -> (w4433:refnum<visa-resource-name>)
                                n4012 = local read "Volume of Syringe"() -> (w4430:dbl)
                                n4013 = call "GoToAbsolutePosition(SubVI).vi"("Absolute Volume Position in Syringe (in ul)"=0.0 ("Volume to be picked up"), "Volume of Syringe"=w4430, "Resolution of Pumping"=T2."Standard Pumping" ("Resolution of PickUP"), "Flow Rate (ul/min)"=150.0 ("PickUp Flow Rate (ul/min)"), "VISA Refnum in"=w4433) -> ()  [unwired: 6 in, 1 out]
                                }
                                frame #7 {
                                n4014 = local read "Stopper that ends \nthe main loops"() -> (w4434:bool)
                                n4015 = local read "VISA Refnum in\nfor Pump"() -> (w4435:refnum<visa-resource-name>)
                                n4016 = case shown="True" w4434 {
                                frame False {
                                }
                                frame True {
                                n4017 = local read "VISA Refnum in\nfor Pump"() -> (w4436:refnum<visa-resource-name>)
                                n4018 = call "HardStopCurrentProcess (SubVI).vi"("VISA Refnum in"=w4436) -> ()  [unwired: 11 in]
                                }
                                }
                                n4019 = call "ProcessCompletionWaiter (SubVI).vi"("VISA Refnum in"=w4435) -> ()  [unwired: 11 in]
                                }
                              }
                              n4020 = local write "Pause Data Collection"(TRUE ("Pause Data Collection")) -> ()
                            }
                          }
                          frame #2 {
                            # "Switch to Port-7"
                            # "Port-7 of pump is connected to Buffer-B"
                            n4021 = local read "VISA Refnum in\nfor Pump"() -> (w4438:refnum<visa-resource-name>)
                            n4022 = local read "Port for \nB-Elution"() -> (w4437:string)
                            n4023 = call "PortChanger (SubVI).vi"("Port Number"=w4437, "VISA Refnum in"=w4438) -> ()  [unwired: 10 in]
                          }
                          frame #3 {
                            n4024 = local read "VISA Refnum in\nfor Pump"() -> (w4439:refnum<visa-resource-name>)
                            n4025 = call "ProcessCompletionWaiter (SubVI).vi"("VISA Refnum in"=w4439) -> ()  [unwired: 11 in]
                          }
                          frame #4 {
                            # "External vale is temporarily connected to teh waste outlet in this code"
                            n4026 = local write "Valve V3 Open"(FALSE ("Valve V3 Open")) -> ()
                            n4027 = local write "Valve V4 Open"(FALSE ("Valve V4 Open")) -> ()
                            n4028 = local write "Valve V1 Open"(FALSE ("Valve V1 Open")) -> ()
                            n4029 = local write "Valve V2 Open"(FALSE ("Valve V2 Open")) -> ()
                            n4030 = local write "External Valve \nOpen"(FALSE ("External Valve \nOpen")) -> ()
                            n4031 = local write "Valve V8 Open"(TRUE ("Valve V8 Open")) -> ()
                            n4032 = local write "Valve V6 Open"(FALSE ("Valve V6 Open")) -> ()
                            n4033 = local write "Valve V5 Open"(FALSE ("Valve V5 Open")) -> ()
                            n4034 = local write "Valve V7 Open"(FALSE ("Valve V7 Open")) -> ()
                          }
                          frame #5 {
                            n4035 = local read "Apparent Volume\nof Syringe"() -> (w4449:dbl)
                            n4036 = local read "Buffer-B Volume \nfor elution tubing \npre-wash"() -> (w4452:dbl)
                            n4037 = Quotient & Remainder(x=w4452, y=w4449) -> (x-y*floor(x/y)=w4450:dbl, floor(x/y)=w4451:dbl)
                            n4038 = for {
                              N: w4451 -> [_]
                              n4039 = stacked-sequence {
                                frame #0 {
                                n4040 = local read "Buffer-B PickUp \nFlow Rate (ul/min)"() -> (w4455:dbl)
                                n4041 = local read "Buffer-B Pumping\nResolution"() -> (w4454:T2)
                                n4042 = local read "VISA Refnum in\nfor Pump"() -> (w4457:refnum<visa-resource-name>)
                                n4043 = local read "Apparent Volume\nof Syringe"() -> (w4453:dbl)
                                n4044 = local read "Volume of Syringe"() -> (w4456:dbl)
                                n4045 = call "RPickUp(SubVI).vi"("Volume to be picked up"=w4453, "Volume of Syringe"=w4456, "Resolution of PickUP"=w4454, "PickUp Flow Rate (ul/min)"=w4455, "VISA Refnum in"=w4457) -> ()  [unwired: 6 in, 1 out]
                                }
                                frame #1 {
                                n4046 = while {
                                stop <- w4458 stop-if-true
                                n4047 = local read "Stopper that ends \nthe main loops"() -> (w4459:bool)
                                n4048 = local read "VISA Refnum in\nfor Pump"() -> (w4460:refnum<visa-resource-name>)
                                n4049 = case shown="True" w4459 {
                                frame False {
                                }
                                frame True {
                                n4050 = local read "VISA Refnum in\nfor Pump"() -> (w4461:refnum<visa-resource-name>)
                                n4051 = call "HardStopCurrentProcess (SubVI).vi"("VISA Refnum in"=w4461) -> ()  [unwired: 11 in]
                                }
                                }
                                n4052 = call "ProcessCompletionWaiterWithOutPut (SubVI).vi"("VISA Refnum in"=w4460) -> ("Boolean"=w4458:bool)  [unwired: 10 in]
                                }
                                }
                                frame #2 {
                                # "Reads the initial Plunger Position for computing the volume dispensed"
                                n4053 = local read "VISA Refnum in\nfor Pump"() -> (w4463:refnum<visa-resource-name>)
                                n4054 = call "AbsolutePlungerPosition (SubVI).vi"("VISA Refnum in"=w4463) -> ("Plunger Position"=w4462:i32)  [unwired: 10 in]
                                n4055 = local write "Initial Plunger Position"(w4462) -> ()
                                }
                                frame #3 {
                                # "Switch to Port-8"
                                # "Port-8 of the pump is conncted to elution tubing for column-1 of chip"
                                n4056 = local read "VISA Refnum in\nfor Pump"() -> (w4465:refnum<visa-resource-name>)
                                n4057 = call "PortChanger (SubVI).vi"("Port Number"="8", "VISA Refnum in"=w4465) -> ()  [unwired: 10 in]
                                }
                                frame #4 {
                                n4058 = while {
                                stop <- w4466 stop-if-true
                                n4059 = local read "Stopper that ends \nthe main loops"() -> (w4467:bool)
                                n4060 = local read "VISA Refnum in\nfor Pump"() -> (w4468:refnum<visa-resource-name>)
                                n4061 = case shown="True" w4467 {
                                frame False {
                                }
                                frame True {
                                n4062 = local read "VISA Refnum in\nfor Pump"() -> (w4469:refnum<visa-resource-name>)
                                n4063 = call "HardStopCurrentProcess (SubVI).vi"("VISA Refnum in"=w4469) -> ()  [unwired: 11 in]
                                }
                                }
                                n4064 = call "ProcessCompletionWaiterWithOutPut (SubVI).vi"("VISA Refnum in"=w4468) -> ("Boolean"=w4466:bool)  [unwired: 10 in]
                                }
                                }
                                frame #5 {
                                n4065 = local read "Buffer-B Dispense\nFlow Rate for Elution \ntubing pre-wash"() -> (w4473:dbl)
                                n4066 = local read "Buffer-B Pumping\nResolution"() -> (w4472:T2)
                                n4067 = local read "VISA Refnum in\nfor Pump"() -> (w4475:refnum<visa-resource-name>)
                                n4068 = local write "Pause Data Collection"(TRUE ("Pause Data Collection")) -> ()
                                n4069 = local read "Volume of Syringe"() -> (w4474:dbl)
                                n4070 = call "GoToAbsolutePosition(SubVI).vi"("Absolute Volume Position in Syringe (in ul)"=0.0, "Volume of Syringe"=w4474, "Resolution of Pumping"=w4472, "Flow Rate (ul/min)"=w4473, "VISA Refnum in"=w4475) -> ()  [unwired: 6 in, 1 out]
                                }
                                frame #6 {
                                n4071 = local read "VISA Refnum in\nfor Pump"() -> (w4479:refnum<visa-resource-name>)
                                n4072 = local read "Initial Plunger Position"() -> (w4478:dbl)
                                n4073 = local read "Volume of Syringe"() -> (w4476:dbl)
                                n4074 = local read "Buffer-B Pumping\nResolution"() -> (w4477:T2)
                                n4075 = while {
                                tunnel: w4478 -> [w4486]
                                tunnel: w4479 -> [w4485]
                                tunnel: w4477 -> [w4484]
                                tunnel: w4476 -> [w4483]
                                stop <- w4481 stop-if-true
                                n4076 = stacked-sequence {
                                tunnel: w4486 -> [w4493 _]
                                tunnel: w4485 -> [w4492 w4513]
                                tunnel: w4484 -> [w4491 _]
                                tunnel: w4483 -> [w4490 _]
                                tunnel: [_ w4511] -> w4481
                                frame #0 {
                                n4077 = call "AbsolutePlungerPosition (SubVI).vi"("VISA Refnum in"=w4492) -> ("Plunger Position"=w4489:i32)  [unwired: 10 in]
                                n4078 = case shown="\"Standard Pumping\", Default" w4491 {
                                tunnel: w4493 -> [w4498 w4507]
                                tunnel: w4489 -> [w4499 w4506]
                                tunnel: [w4497 w4504] -> w4488
                                tunnel: w4490 -> [w4496 w4505]
                                frame "Standard Pumping", Default {
                                n4079 = Subtract(x=w4498, y=w4499) -> (x-y=w4495:dbl)
                                n4080 = Absolute Value(x=w4495) -> (abs(x)=w4494:dbl)
                                n4081 = Multiply(x=w4494, y=w4496) -> (x*y=w4501:dbl)
                                n4082 = Divide(x=w4501, y=3000.0) -> (x/y=w4497:dbl)
                                }
                                frame "High Resolution Pumping" {
                                n4083 = Subtract(x=w4507, y=w4506) -> (x-y=w4503:dbl)
                                n4084 = Absolute Value(x=w4503) -> (abs(x)=w4502:dbl)
                                n4085 = Multiply(x=w4502, y=w4505) -> (x*y=w4509:dbl)
                                n4086 = Divide(x=w4509, y=24000.0) -> (x/y=w4504:dbl)
                                }
                                }
                                n4087 = local write "Volume being Injected \nin this process"(w4488) -> ()
                                }
                                frame #1 {
                                n4088 = call "LSPOneStatus (SubVI).vi"("VISA Refnum in"=w4513) -> ("read buffer"=w4515:string)  [unwired: 10 in]
                                n4089 = call <vilib>:"Trim Whitespace.vi"("string"=w4515) -> ("trimmed string"=w4514:string)  [unwired: 1 in]
                                n4090 = local read "Stopper that ends \nthe main loops"() -> (w4510:bool)
                                n4091 = Equal?(x=w4514, y="/0`\u0003") -> (x = y?=w4512:bool)
                                n4092 = Or(x=w4512, y=w4510) -> (x .or. y?=w4511:bool)
                                }
                                }
                                n4093 = Wait (ms)(milliseconds to wait=u32 100) -> ()  [unwired: 1 out]
                                n4094 = local read "Stopper that ends \nthe main loops"() -> (w4480:bool)
                                n4095 = case shown="True" w4480 {
                                frame False {
                                }
                                frame True {
                                n4096 = local read "VISA Refnum in\nfor Pump"() -> (w4487:refnum<visa-resource-name>)
                                n4097 = call "HardStopCurrentProcess (SubVI).vi"("VISA Refnum in"=w4487) -> ()  [unwired: 11 in]
                                }
                                }
                                }
                                }
                                frame #7 {
                                # "Change the pump port back to Buffer-B"
                                n4098 = local read "VISA Refnum in\nfor Pump"() -> (w4518:refnum<visa-resource-name>)
                                n4099 = local read "Port for \nB-Elution"() -> (w4517:string)
                                n4100 = local write "Pause Data Collection"(TRUE ("Pause Data Collection")) -> ()
                                n4101 = Wait (ms)(milliseconds to wait=u32 500) -> ()  [unwired: 1 out]
                                n4102 = call "PortChanger (SubVI).vi"("Port Number"=w4517, "VISA Refnum in"=w4518) -> ()  [unwired: 10 in]
                                }
                                frame #8 {
                                n4103 = local read "VISA Refnum in\nfor Pump"() -> (w4521:refnum<visa-resource-name>)
                                n4104 = local write "Volume being Injected \nin this process"(0.0 ("Volume being Injected \nin this process")) -> ()
                                n4105 = call "ProcessCompletionWaiter (SubVI).vi"("VISA Refnum in"=w4521) -> ()  [unwired: 11 in]
                                }
                              }
                            }
                            n4106 = local write "Reminder of the \nVolume to be \nPumped"(w4450) -> ()
                          }
                          frame #6 {
                            n4107 = stacked-sequence {
                              frame #0 {
                                n4108 = local read "Buffer-B PickUp \nFlow Rate (ul/min)"() -> (w4525:dbl)
                                n4109 = local read "Buffer-B Pumping\nResolution"() -> (w4524:T2)
                                n4110 = local read "VISA Refnum in\nfor Pump"() -> (w4527:refnum<visa-resource-name>)
                                n4111 = local read "Reminder of the \nVolume to be \nPumped"() -> (w4523:dbl)
                                n4112 = local read "Volume of Syringe"() -> (w4526:dbl)
                                n4113 = call "RPickUp(SubVI).vi"("Volume to be picked up"=w4523, "Volume of Syringe"=w4526, "Resolution of PickUP"=w4524, "PickUp Flow Rate (ul/min)"=w4525, "VISA Refnum in"=w4527) -> ()  [unwired: 6 in, 1 out]
                              }
                              frame #1 {
                                n4114 = while {
                                stop <- w4528 stop-if-true
                                n4115 = local read "Stopper that ends \nthe main loops"() -> (w4529:bool)
                                n4116 = local read "VISA Refnum in\nfor Pump"() -> (w4530:refnum<visa-resource-name>)
                                n4117 = case shown="True" w4529 {
                                frame False {
                                }
                                frame True {
                                n4118 = local read "VISA Refnum in\nfor Pump"() -> (w4531:refnum<visa-resource-name>)
                                n4119 = call "HardStopCurrentProcess (SubVI).vi"("VISA Refnum in"=w4531) -> ()  [unwired: 11 in]
                                }
                                }
                                n4120 = call "ProcessCompletionWaiterWithOutPut (SubVI).vi"("VISA Refnum in"=w4530) -> ("Boolean"=w4528:bool)  [unwired: 10 in]
                                }
                              }
                              frame #2 {
                                # "Reads the initial Plunger Position for computing the volume dispensed"
                                n4121 = local read "VISA Refnum in\nfor Pump"() -> (w4533:refnum<visa-resource-name>)
                                n4122 = call "AbsolutePlungerPosition (SubVI).vi"("VISA Refnum in"=w4533) -> ("Plunger Position"=w4532:i32)  [unwired: 10 in]
                                n4123 = local write "Initial Plunger Position"(w4532) -> ()
                              }
                              frame #3 {
                                # "Switch to Port-8"
                                # "Port-8 of the pump is conncted to elution inlet of column-1 of chip"
                                n4124 = local read "VISA Refnum in\nfor Pump"() -> (w4535:refnum<visa-resource-name>)
                                n4125 = call "PortChanger (SubVI).vi"("Port Number"="8", "VISA Refnum in"=w4535) -> ()  [unwired: 10 in]
                              }
